vi "Check Action.vi"(6 "HRS Time":dbl, 7 "Values In":dbl[](array[numeric]), 8 "error in (no error)":errorcluster, 11 "Valve in":refnum<class "ValueSetControl.lvclass">) -> (0 "error out":errorcluster, 1 "Do Action":bool, 2 "Action":T1, 3 "Valve out":refnum<class "ValueSetControl.lvclass">, 5 "Values":dbl[](array[numeric]))   [LabVIEW 2020, in "VolatusControl.lvlib" / "ValueSetControl.lvclass"]
uses:
  ValueSetControl.lvclass
  ValueSetControl.lvclass/ValueSetControl.ctl
  lv-vecto/Vecto/Vecto.lvlib
  Volatus/MessageQ/MessageQ.lvclass
  Valve Action.ctl
  VolatusControl.lvlib
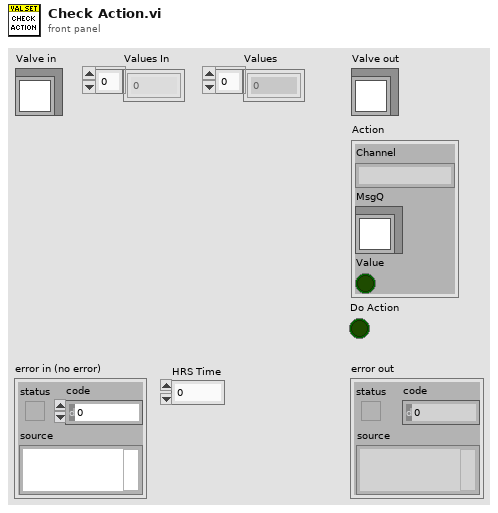
[diagram p1: front panel]
types:
  T1 = typedef "VolatusControl.lvlib/Valve Action.ctl" = cluster{"Channel":string, "MsgQ":refnum<class "MessageQ.lvclass">, "Value":bool}
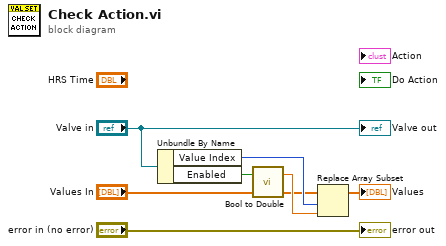
[diagram p0: block diagram]
diagram:
  n1 = Unbundle By Name("Valve in") -> ("Value Index"=w5:i32, "Enabled"=w6:bool)
  n2 = call "Bool to Double.vi"("Bool"=w6) -> ("Double"=w4:dbl)  [unwired: 2 in]
  n3 = Replace Array Subset(array="Values In", new element=w4, index=w5) -> (→"Values":dbl[])
  "error out" <- "error in (no error)"
  "Valve out" <- "Valve in"
